vi "TCPIP Communication.vi"() -> ()   [LabVIEW 2018]
uses:
  RxTx/RxTx.lvclass
panel:
  in  "Remote IP":string
  out "error out 6":errorcluster
  out "error out 4":errorcluster
  out "error out 5":errorcluster
  in  "RxTx in 2":refnum<class "RxTx.lvclass">
  in  "RxTx in":refnum<class "RxTx.lvclass">
  # "Filter Wheel Communication System"
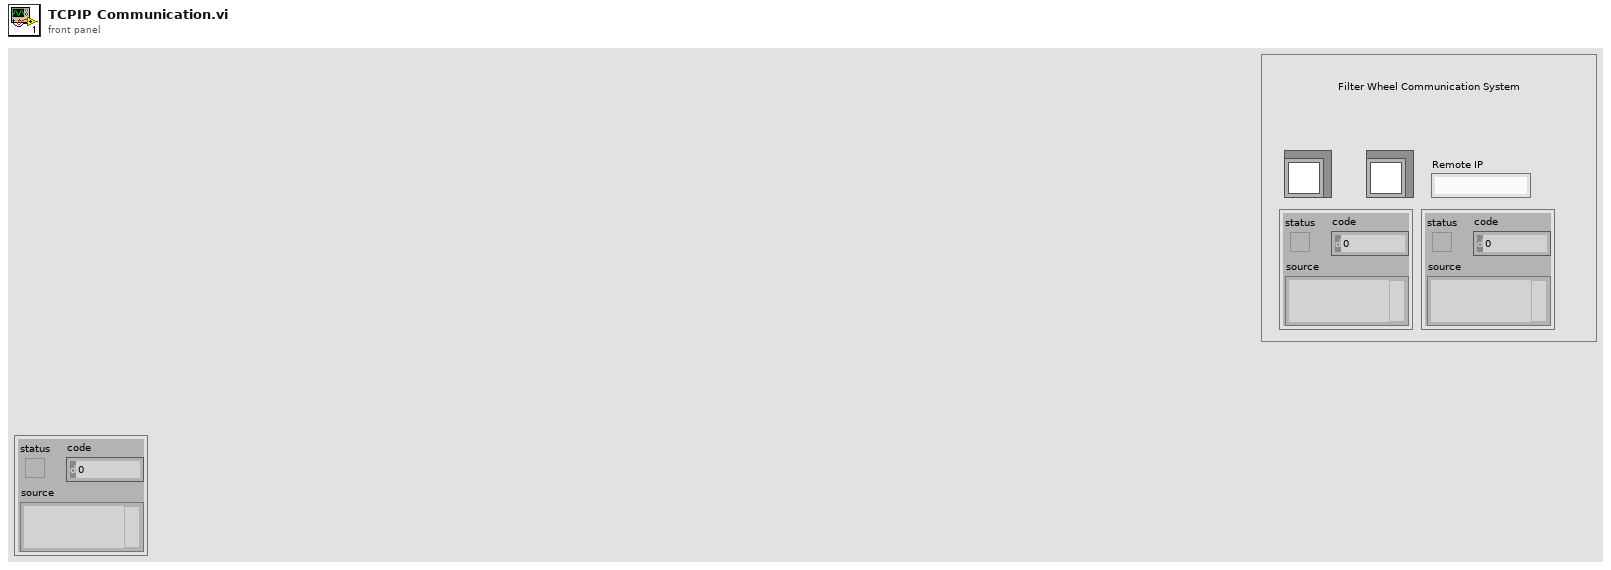
[diagram p1: front panel]
types:
  T1 = enum16{"Standard", "Buffered", "CRLF", "Immediate"}
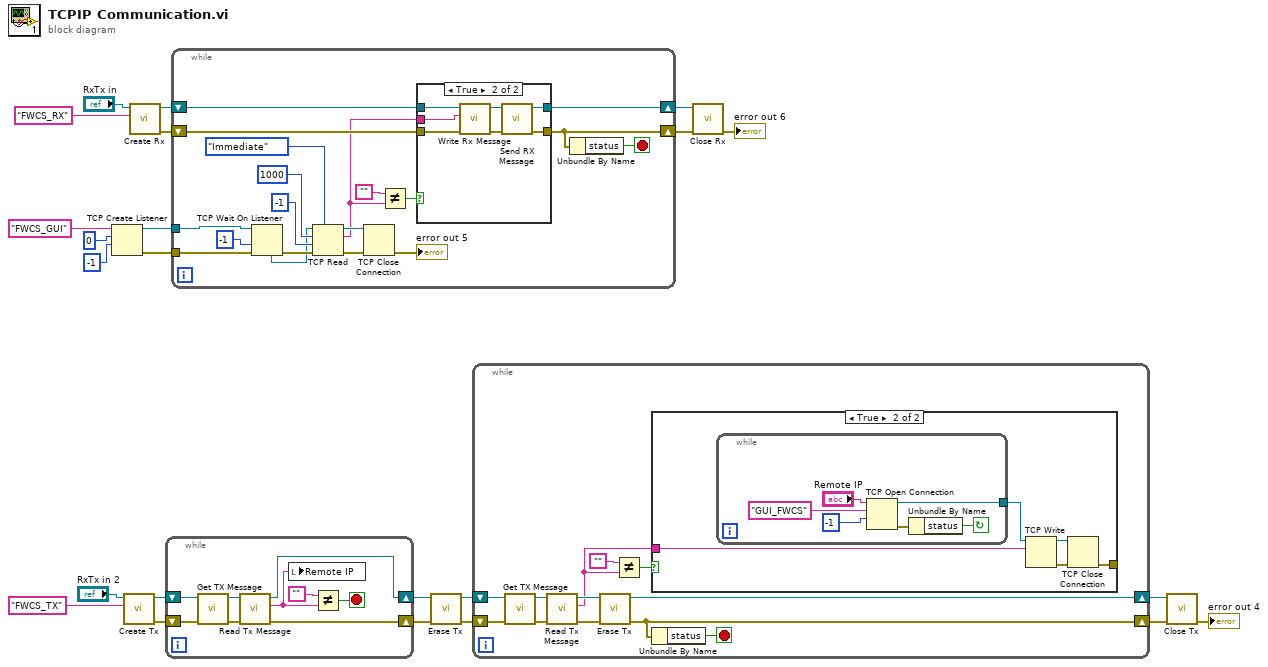
[diagram p0: block diagram]
diagram:
  n1 = TCP Create Listener(9:-1 ("timeout ms (25000)"), 10:u16 0 ("port"), 11:"FWCS_GUI" ("service name")) -> (0:w5:errorcluster, 3:w4:refnum<k5>)  [unwired: 2 in, 1 out]
  n2 = call "Create Tx.vi"("Writer Name"="FWCS_TX" ("Reader Name"), "RxTx in"="RxTx in 2") -> ("error out"=w12:errorcluster, "RxTx out"=w13:refnum<class "RxTx.lvclass">)  [unwired: 8 in]
  n3 = call "Create Rx.vi"("Reader Name"="FWCS_RX", "RxTx in"="RxTx in") -> ("error out"=w22:errorcluster, "RxTx out"=w23:refnum<class "RxTx.lvclass">)  [unwired: 8 in]
  n4 = while {
    shift-right: [w25] -> w11
    shift-left: w13 -> [w28]
    shift-right: [w26] -> w8
    shift-left: w12 -> [w27]
    stop <- w29 stop-if-true
    n5 = call "Get TX Message.vi"("error in (no error)"=w27, "RxTx in"=w28) -> ("error out"=w30:errorcluster, "RxTx out"=w31:refnum<class "RxTx.lvclass">)  [unwired: 8 in]
    n6 = call "Read Tx Message.vi"("error in (no error)"=w30, "RxTx in"=w31) -> ("error out"=w26:errorcluster, "Tx Message"=w24:string, "RxTx out"=w25:refnum<class "RxTx.lvclass">)  [unwired: 7 in]
    n7 = local write "Remote IP"(w24) -> ()
    n8 = Not Equal?(x="", y=w24) -> (x != y?=w29:bool)
  }
  n9 = while {
    shift-right: [w49] -> w20
    shift-left: w23 -> [w51]
    shift-right: [w45] -> w21
    shift-left: w22 -> [w50]
    tunnel: w5 -> [w34]
    tunnel: w4 -> [w33]
    stop <- w48 stop-if-true
    n10 = TCP Wait On Listener(8:w34, 9:-1 ("timeout ms (wait forever: -1)"), 11:w33) -> (0:w40:errorcluster, 4:w36:refnum<k5>)  [unwired: 1 in, 3 out]
    n11 = TCP Read(connection ID=w36, bytes to read=1000, error in (no error)=w40, 7:T1."Immediate" ("mode (standard)"), 9:-1 ("timeout ms (25000)")) -> (connection ID out=w38:refnum<k5>, data out=w35:string, error out=w37:errorcluster)
    n12 = TCP Close Connection(connection ID=w38, error in (no error)=w37) -> (error out=→"error out 5":errorcluster)  [unwired: 1 in, 1 out]
    n13 = Not Equal?(x="", y=w35) -> (x != y?=w47:bool)
    n14 = case shown="True" w47 {
      tunnel: w51 -> [w53 w60]
      tunnel: w50 -> [w52 w59]
      tunnel: [w53 w56] -> w49
      tunnel: [w52 w55] -> w45
      tunnel: w35 -> [_ w54]
      frame False {
      }
      frame True {
        n15 = call "Write Rx Message.vi"("error in (no error)"=w59, "Rx Message"=w54, "RxTx in"=w60) -> ("error out"=w58:errorcluster, "RxTx out"=w57:refnum<class "RxTx.lvclass">)  [unwired: 7 in]
        n16 = call "Send RX Message.vi"("error in (no error)"=w58, "RxTx in"=w57) -> ("error out"=w55:errorcluster, "RxTx out"=w56:refnum<class "RxTx.lvclass">)  [unwired: 8 in]
      }
    }
    n17 = Unbundle By Name(w45) -> ("status"=w48:bool)
  }
  n18 = call "Erase Tx.vi"("error in (no error)"=w8, "RxTx in"=w11) -> ("error out"=w9:errorcluster, "RxTx out"=w10:refnum<class "RxTx.lvclass">)  [unwired: 8 in]
  n19 = while {
    shift-right: [w67] -> w18
    shift-left: w10 -> [w65]
    shift-right: [w64] -> w19
    shift-left: w9 -> [w66]
    stop <- w63 stop-if-true
    n20 = call "Get TX Message.vi"("error in (no error)"=w66, "RxTx in"=w65) -> ("error out"=w72:errorcluster, "RxTx out"=w71:refnum<class "RxTx.lvclass">)  [unwired: 8 in]
    n21 = call "Read Tx Message.vi"("error in (no error)"=w72, "RxTx in"=w71) -> ("error out"=w70:errorcluster, "Tx Message"=w62:string, "RxTx out"=w69:refnum<class "RxTx.lvclass">)  [unwired: 7 in]
    n22 = call "Erase Tx.vi"("error in (no error)"=w70, "RxTx in"=w69) -> ("error out"=w64:errorcluster, "RxTx out"=w67:refnum<class "RxTx.lvclass">)  [unwired: 8 in]
    n23 = Not Equal?(x="", y=w62) -> (x != y?=w61:bool)
    n24 = case shown="True" w61 {
      tunnel: w62 -> [_ w77]
      tunnel: [_ w74] -> _
      frame False {
      }
      frame True {
        n25 = while {
          tunnel: [w80] -> w76
          stop <- w83 continue-if-true
          n26 = TCP Open Connection(address="Remote IP", remote port or service name="GUI_FWCS", timeout ms (60000)=-1 ("timeout")) -> (connection ID=w80:refnum<k5>, error out=w82:errorcluster)  [unwired: 2 in]
          n27 = Unbundle By Name(w82) -> ("status"=w83:bool)
        }
        n28 = TCP Write(connection ID=w76, data in=w77) -> (connection ID out=w73:refnum<k5>, error out=w75:errorcluster)  [unwired: 2 in, 1 out]
        n29 = TCP Close Connection(connection ID=w73, error in (no error)=w75) -> (error out=w74:errorcluster)  [unwired: 1 in, 1 out]
      }
    }
    n30 = Unbundle By Name(w64) -> ("status"=w63:bool)
  }
  n31 = call "Close Rx.vi"("error in (no error)"=w21, "RxTx in"=w20) -> ("error out"=→"error out 6":errorcluster)  [unwired: 8 in, 1 out]
  n32 = call "Close Tx.vi"("error in (no error)"=w19, "RxTx in"=w18) -> ("error out"=→"error out 4":errorcluster)  [unwired: 8 in, 1 out]
